vi "10 s time subvi.vi"(10 "Under/ Air TimeElapsed":dbl, 11 "Under/Air":dbl) -> (2 "Numeric 2":dbl, 3 "Numeric":dbl)   [LabVIEW 2019]
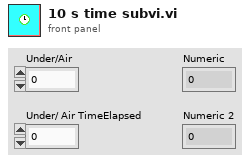
[diagram p1: front panel]
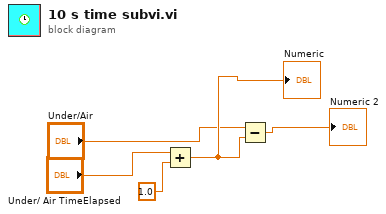
[diagram p0: block diagram]
diagram:
  n1 = Add(x="Under/ Air TimeElapsed", y=1.0) -> (x+y=w5:dbl)
  "Numeric" <- w5
  n2 = Subtract(x="Under/Air", y=w5) -> (x-y=→"Numeric 2":dbl)
